vi "4. 藍幕電影.vi"() -> ()   [LabVIEW 2014]
uses:
  <vilib>/vision/NI_Vision_Development_Module.lvlib
  <vilib>/vision/driver/NI_Vision_Acquisition_Software.lvlib
panel:
  out "appended path":path
  in  "開始錄影":bool
  out "Thresholded Image":T1(plugin-control) caption="HSL Threshold"
  out "Image":T1(plugin-control)
  in  "亮度":cluster{"Min":i32, "Max":i32}(slide)={"Min"=60, "Max"=157} scale=0.0..255.0
  in  "飽和度":cluster{"Min":i32, "Max":i32}(slide)={"Min"=0, "Max"=42} scale=0.0..255.0
  in  "色相":cluster{"Min":i32, "Max":i32}(slide)={"Min"=67, "Max"=120} scale=0.0..255.0
  in  "停止":bool
  out "Thresholded Image 2":T1(plugin-control) caption="HSL Threshold"
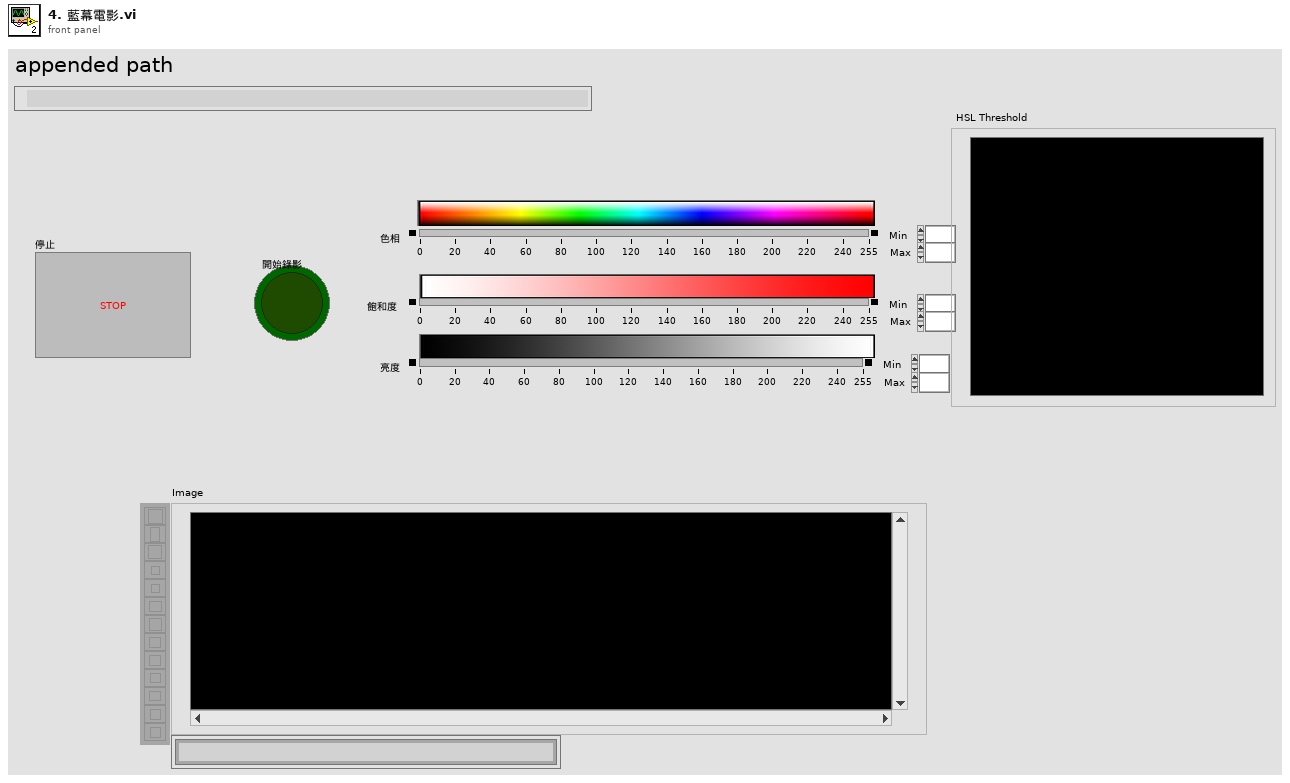
[diagram p1: front panel]
types:
  T1 = typedef "IMAQ Image.ctl" = refnum<image>
  T2 = typedef "Image Type" = u32
  T3 = cluster{"Type":u32, "Version":u32, "Flags":u32, "SerialNumberHigh":u32, "SerialNumberLow":u32, "BusType":u32, "InterfaceName":string, "VendorName":string, "ModelName":string, "CameraFileName":string, "CameraAttributeURL":string}[]
  T4 = cluster{"Type":u32, "Version":u32, "Flags":u32, "SerialNumberHigh":u32, "SerialNumberLow":u32, "BusType":u32, "InterfaceName":string, "VendorName":string, "ModelName":string, "CameraFileName":string, "CameraAttributeURL":string}
  T5 = typedef "IMAQdx.ctl" = refnum<k21>
  T6 = typedef "AviRefnum.ctl" = refnum<k1>
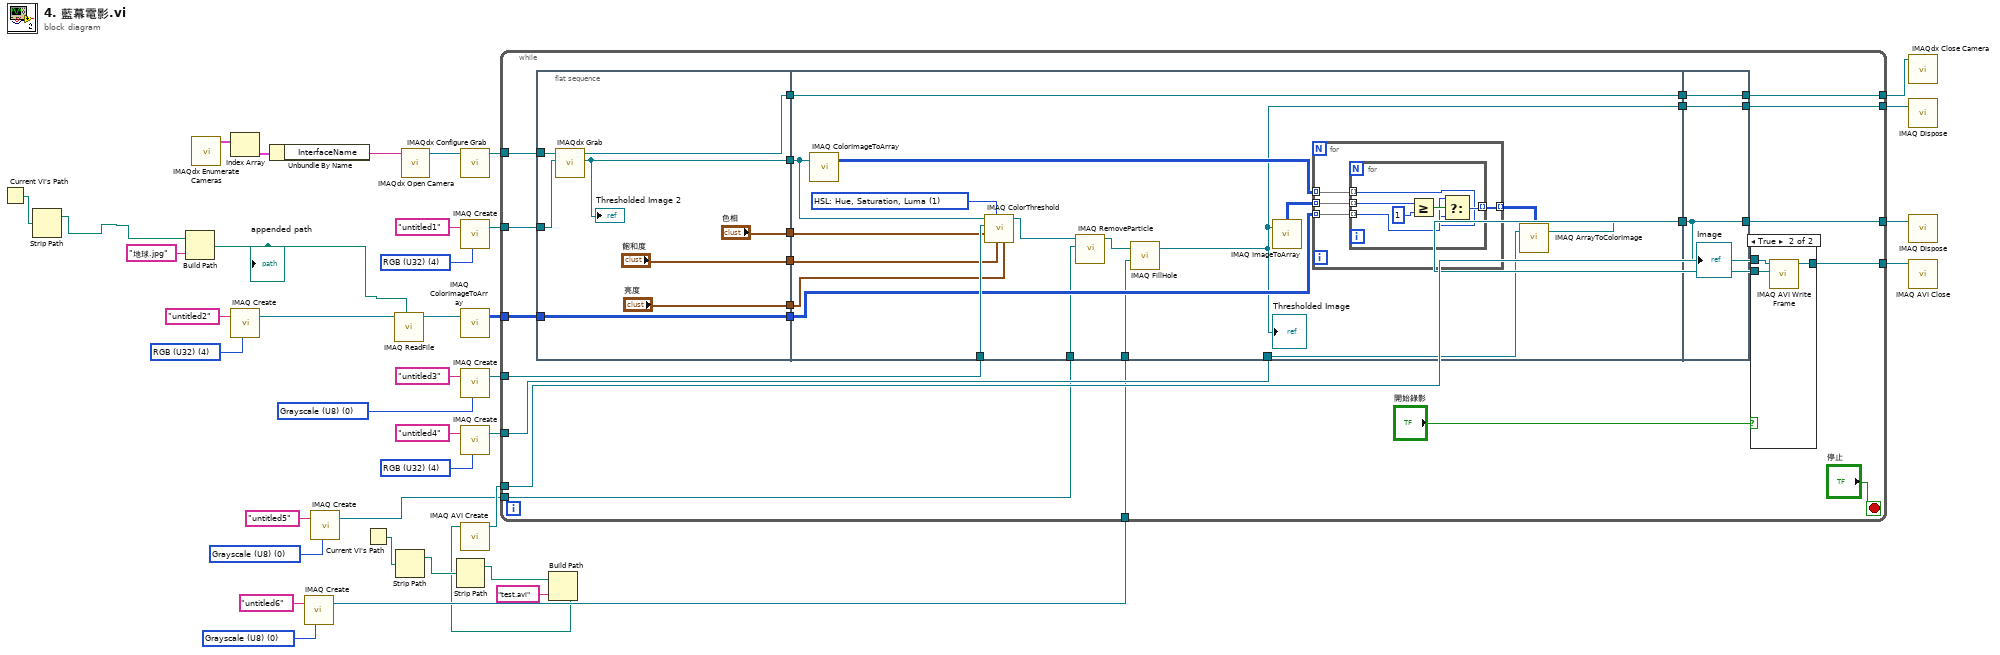
[diagram p0: block diagram]
diagram:
  w14 = T2 0 items=["Grayscale (U8)", "Grayscale (I16)", "Grayscale (SGL)", "Complex (CSG)", "RGB (U32)", "HSL (U32)", "RGB (U64)", "Grayscale (U16)"] ("Image Type")
  w15 = T2 0 items=["Grayscale (U8)", "Grayscale (I16)", "Grayscale (SGL)", "Complex (CSG)", "RGB (U32)", "HSL (U32)", "RGB (U64)", "Grayscale (U16)"] ("Image Type")
  w21 = T2 4 items=["Grayscale (U8)", "Grayscale (I16)", "Grayscale (SGL)", "Complex (CSG)", "RGB (U32)", "HSL (U32)", "RGB (U64)", "Grayscale (U16)"] ("Image Type")
  w25 = T2 4 items=["Grayscale (U8)", "Grayscale (I16)", "Grayscale (SGL)", "Complex (CSG)", "RGB (U32)", "HSL (U32)", "RGB (U64)", "Grayscale (U16)"] ("Image Type")
  w30 = T2 0 items=["Grayscale (U8)", "Grayscale (I16)", "Grayscale (SGL)", "Complex (CSG)", "RGB (U32)", "HSL (U32)", "RGB (U64)", "Grayscale (U16)"] ("Image Type")
  w31 = T2 4 items=["Grayscale (U8)", "Grayscale (I16)", "Grayscale (SGL)", "Complex (CSG)", "RGB (U32)", "HSL (U32)", "RGB (U64)", "Grayscale (U16)"] ("Image Type")
  n1 = Current VI's Path() -> (path=w4:path)
  n2 = Strip Path(path=w4) -> (stripped path=w1:path)  [unwired: 1 out]
  n3 = Build Path(base path=w1, name or relative path="地球.jpg") -> (appended path=w3:path)
  "appended path" <- w3
  n4 = call <vilib>:"IMAQdx Enumerate Cameras.vi"() -> ("Camera Information Array"=w39:T3)  [unwired: 10 in, 1 out]
  n5 = Index Array(array=w39) -> (element=w38:T4)  [unwired: 1 in]
  n6 = call "IMAQ Create"("Image Name"="untitled2", "Image Type"=w21) -> ("New Image"=w19:T1)  [unwired: 3 in, 1 out]
  n7 = Unbundle By Name(w38) -> ("InterfaceName"=w37:string)
  n8 = call "IMAQ Create"("Image Name"="untitled6", "Image Type"=w14) -> ("New Image"=w10:T1)  [unwired: 3 in, 1 out]
  n9 = call "IMAQ Create"("Image Name"="untitled5", "Image Type"=w15) -> ("New Image"=w11:T1)  [unwired: 3 in, 1 out]
  n10 = Current VI's Path() -> (path=w9:path)
  n11 = call "IMAQ ReadFile"("File Path"=w3, "Image"=w19) -> ("Image Out"=w18:T1)  [unwired: 5 in, 4 out]
  n12 = Strip Path(path=w9) -> (stripped path=w8:path)  [unwired: 1 out]
  n13 = call <vilib>:"IMAQdx Open Camera.vi"("Session In"=w37) -> ("Session Out"=w36:T5)  [unwired: 9 in, 1 out]
  n14 = Strip Path(path=w8) -> (stripped path=w7:path)  [unwired: 1 out]
  n15 = call <vilib>:"IMAQdx Configure Grab.vi"("Session In"=w36) -> ("Session Out"=w35:T5)  [unwired: 9 in, 1 out]
  n16 = call "IMAQ Create"("Image Name"="untitled1", "Image Type"=w31) -> ("New Image"=w32:T1)  [unwired: 3 in, 1 out]
  n17 = call "IMAQ ColorImageToArray"("Image"=w18) -> ("Image Pixels (U32)"=w17:u32[][])  [unwired: 3 in, 2 out]
  n18 = call "IMAQ Create"("Image Name"="untitled3", "Image Type"=w30) -> ("New Image"=w28:T1)  [unwired: 3 in, 1 out]
  n19 = call "IMAQ Create"("Image Name"="untitled4", "Image Type"=w25) -> ("New Image"=w24:T1)  [unwired: 3 in, 1 out]
  n20 = Build Path(base path=w7, name or relative path="test.avi") -> (appended path=w5:path)
  n21 = call "IMAQ AVI Create"("AVI Path"=w5) -> ("Avi Refnum"=w16:T6)  [unwired: 9 in, 1 out]
  n22 = while {
    tunnel: w35 -> [w62]
    tunnel: [w59] -> w34
    tunnel: w32 -> [w58]
    tunnel: w28 -> [w57]
    tunnel: [w53] -> w27
    tunnel: w24 -> [w51]
    tunnel: [w43] -> w23
    tunnel: [w44] -> w22
    tunnel: w17 -> [w46]
    tunnel: w16 -> [w45]
    tunnel: w11 -> [w41]
    tunnel: w10 -> [w40]
    stop <- "停止" stop-if-true
    n23 = flat-sequence {
      tunnel: w62 -> [w74]
      tunnel: [w73] -> w61
      tunnel: [w68] -> w60
      tunnel: w58 -> [w72]
      tunnel: ["色相"] -> w56
      tunnel: ["飽和度"] -> w55
      tunnel: ["亮度"] -> w54
      tunnel: [w67] -> w47
      tunnel: w46 -> [w67]
      tunnel: w61 -> [w91]
      tunnel: w60 -> [w85]
      tunnel: w57 -> [w90]
      tunnel: w56 -> [w89]
      tunnel: w55 -> [w88]
      tunnel: w54 -> [w87]
      tunnel: w51 -> [w83]
      tunnel: [w91] -> w50
      tunnel: [w77] -> w49
      tunnel: [w82] -> w48
      tunnel: w47 -> [w81]
      tunnel: w41 -> [w76]
      tunnel: w40 -> [w75]
      tunnel: w50 -> [w105]
      tunnel: w49 -> [w104]
      tunnel: w48 -> [w103]
      tunnel: [w105] -> w59
      tunnel: [w104] -> w53
      tunnel: [w103] -> w43
      frame #0 {
        n24 = call <vilib>:"IMAQdx Grab.vi"("Image In"=w72, "Session In"=w74) -> ("Image Out"=w68:T1, "Session Out"=w73:T5)  [unwired: 6 in, 2 out]
        "Thresholded Image 2" <- w68
      }
      frame #1 {
        w92 = 1 items=["RGB (Red, Green, Blue)", "HSL: Hue, Saturation, Luma"] ("Threshold Color Mode")
        n25 = call "IMAQ ColorImageToArray"("Image"=w85) -> ("Image Pixels (U32)"=w86:u32[][])  [unwired: 3 in, 2 out]
        n26 = call "IMAQ ColorThreshold"("Blue or Luma or Val or Inten Range"=w87, "Green or Sat Range"=w88, "Color Mode"=w92, "Red or Hue Range"=w89, "Image Dst"=w90, "Image Src"=w85) -> ("Image Dst Out"=w79:T1)  [unwired: 2 in, 3 out]
        n27 = call "IMAQ RemoveParticle"("Image Dst"=w76, "Image Src"=w79) -> ("Image Dst Out"=w78:T1)  [unwired: 8 in, 1 out]
        n28 = call "IMAQ FillHole"("Image Dst"=w75, "Image Src"=w78) -> ("Image Dst Out"=w77:T1)  [unwired: 4 in, 1 out]
        "Thresholded Image" <- w77
        n29 = call "IMAQ ImageToArray"("Image"=w77) -> ("Image Pixels (U8)"=w84:u8[][])  [unwired: 3 in, 4 out]
        n30 = for {
          tunnel: w84 -> [w96] mode=indexing
          tunnel: w86 -> [w95] mode=indexing
          tunnel: [w94] -> w80 mode=indexing
          tunnel: w81 -> [w93] mode=indexing
          n31 = for {
            tunnel: w96 -> [w99] mode=indexing
            tunnel: w95 -> [w97] mode=indexing
            tunnel: [w102] -> w94 mode=indexing
            tunnel: w93 -> [w98] mode=indexing
            n32 = Greater Or Equal?(x=w99, y=u8 1) -> (x >= y?=w100:bool)
            n33 = Select(t=w98, s=w100, f=w97) -> (s? t:f=w102:u32)
          }
        }
        n34 = call "IMAQ ArrayToColorImage"("Image Pixels (U32)"=w80, "Image"=w83) -> ("Image Out"=w82:T1)  [unwired: 3 in, 1 out]
      }
      frame #2 {
        "Image" <- w103
      }
    }
    n35 = case shown="True" "開始錄影" {
      tunnel: w45 -> [w63 w66]
      tunnel: [w63 w65] -> w44
      tunnel: w43 -> [_ w64]
      frame False {
      }
      frame True {
        n36 = call "IMAQ AVI Write Frame"("Image"=w64, "Avi Refnum"=w66) -> ("Avi Refnum (duplicate)"=w65:T6)  [unwired: 8 in, 1 out]
      }
    }
  }
  n37 = call <vilib>:"IMAQdx Close Camera.vi"("Session In"=w34) -> ()  [unwired: 10 in, 1 out]
  n38 = call "IMAQ Dispose"("Image"=w27) -> ()  [unwired: 5 in, 1 out]
  n39 = call "IMAQ Dispose"("Image"=w23) -> ()  [unwired: 5 in, 1 out]
  n40 = call "IMAQ AVI Close"("Avi Refnum"=w22) -> ()  [unwired: 10 in, 1 out]
